vi "Get Process Model.vi"(8 "error in (no error)":errorcluster, 11 "Execution in":refnum<class "Execution.lvclass">) -> (0 "error out":errorcluster, 2 "Process Model":refnum<class "SequenceFile.lvclass">, 3 "Execution out":refnum<class "Execution.lvclass">)   [LabVIEW 2020, in "TSnax.lvlib" / "Execution.lvclass"]
uses:
  Execution.lvclass
  Execution.lvclass/Execution.ctl
  PropertyObject/PropertyObject.lvclass
  SequenceFile/SequenceFile.lvclass
  C:/dev/illuminated-g/tsnax/TSnax/PropertyObjectFile/PropertyObjectFile.lvclass
  C:/dev/illuminated-g/tsnax/TSnax/PropertyObject/PropertyObject.lvclass
  C:/dev/illuminated-g/tsnax/TSnax/SequenceFile/SequenceFile.lvclass
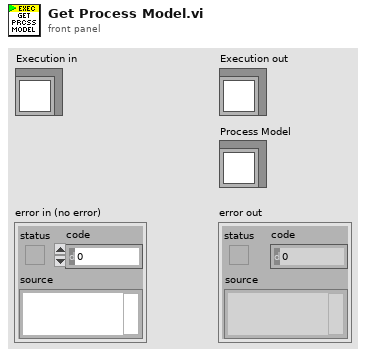
[diagram p1: front panel]
types:
  T1 = typedef "TSnax.lvlib/Execution.lvclass/Ref Data.ctl" = cluster{"Parameters":refnum<class "PropertyObject.lvclass">, "Client Sequence":refnum<class "SequenceFile.lvclass">, "Process Model":refnum<class "SequenceFile.lvclass">, "Entry Sequence":string, "Execution":refnum<k7>, "Report":refnum<class "Report.lvclass">, "Options":T2}
  T2 = typedef "TSnax.lvlib/Execution.lvclass/Execution Options.ctl" = cluster{"Use Default Model":bool, "Release Related Sessions":bool}
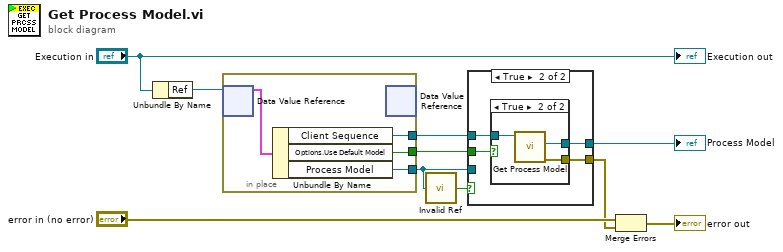
[diagram p0: block diagram]
diagram:
  n1 = Unbundle By Name("Execution in") -> ("Ref"=w9:refnum<data-value>)
  n2 = in-place {
    in-place-border: [w13] -> w4
    in-place-border: [w12] -> w6
    in-place-border: [w11] -> w7
    n3 = in-place-dvr #1(w9) -> (w14:T1)  [unwired: 1 out]
    n4 = Unbundle By Name(w14) -> ("Client Sequence"=w13:refnum<class "SequenceFile.lvclass">, "Options.Use Default Model"=w12:bool, "Process Model"=w11:refnum<class "SequenceFile.lvclass">)
    n5 = in-place-dvr #1() -> ()  [unwired: 1 in, 2 out]
  }
  n6 = call "Invalid Ref.vi"("PropertyObject"=w7) -> ("Not a Valid Ref?"=w5:bool)
  n7 = case shown="True" w5 {
    tunnel: w7 -> [w15 _]
    tunnel: w6 -> [_ w19]
    tunnel: w4 -> [_ w18]
    tunnel: [w15 w17] -> w3
    tunnel: [_ w16] -> w1
    frame False {
    }
    frame True {
      n8 = case shown="True" w19 {
        tunnel: w18 -> [_ w22]
        tunnel: [_ w21] -> w17
        tunnel: [_ w20] -> w16
        frame False {
        }
        frame True {
          n9 = call "Get Process Model.vi"("SequenceFile in"=w22) -> ("error out"=w20:errorcluster, "Process Model"=w21:refnum<class "SequenceFile.lvclass">)  [unwired: 8 in, 1 out]
        }
      }
    }
  }
  "Process Model" <- w3
  n10 = Merge Errors("error in (no error)", w1) -> (→"error out":errorcluster)
  "Execution out" <- "Execution in"
